vi "LEP_RV_BuildSettingsDefault.vi"(3 "error in (no error)":errorcluster) -> (0 "error out":errorcluster, 1 "Default Values":refnum<vi>[](array[refnum]), 2 "Attribute Name":string[](array[string]))   [LabVIEW 2011]
doc: "Sets the default project settings for new LabVIEW Embedded Projects."
uses:
  LEP_RV_Config.ctl
panel:
  in  "Default":T1={"Enable debugging"=TRUE, "Debug Options"=0, "Use stack variables"=FALSE, "Generate serial only"=FALSE, "Generate guard code"=TRUE, "Generate Integer Only"=FALSE, "Generate C Function Calls"=FALSE, "ExpressionFolding"=FALSE, "Constant Allocation"=0, "Constant Deallocation"=0, "Build Specification ID"="", "Preprocessor symbols (define)"="", "Compiler Flags"="", "Linker Flags"="", "Mode"=1, "Optimization"=2, "Optimize for time"=FALSE, "Enable cross-module optimization"=TRUE, "Include paths"=[], "Optimize heap size"=TRUE, "Use MicroLib"=FALSE, "Debug Mode"=2, "Enable profile information"=FALSE, "Host name"="board", "Use DHCP"=TRUE, "IP address"="0.0.0.0", "Subnet mask"="0.0.0.0", "Gateway"="0.0.0.0", "Primary DNS"="0.0.0.0", "Secondary DNS"="0.0.0.0", "MAC in target memory"=TRUE, "MAC address"="", "Console output"=0, "Target serial port"=0} {"Constant Deallocation" items=["Out of Scope", "VI End", "Application End"]; "Constant Allocation" items=["First Use", "Containing Loop", "VI Initialization", "Application Initialization"]; "Target serial port" items=["0", "1", "2", "3"]; "Console output" items=["Processor status window", "Serial port"]; "Optimization" items=["Level 0 (-O0)", "Level 1 (-O1)", "Level 2 (-O2)", "Level 3 (-O3)"]; "Mode" items=["ARM-Mode", "Thumb-Mode"]; "Debug Options" items=["Use ULINK Debugger", "Use Simulator"]; "Debug Mode" items=["Instrumented (serial port)", "Instrumented (TCP/IP)", "Non-instrumented (JTAG/USB)"]}
  out "Default":T1={"Enable debugging"=TRUE, "Debug Options"=0, "Use stack variables"=FALSE, "Generate serial only"=FALSE, "Generate guard code"=TRUE, "Generate Integer Only"=FALSE, "Generate C Function Calls"=FALSE, "ExpressionFolding"=FALSE, "Constant Allocation"=0, "Constant Deallocation"=0, "Build Specification ID"="", "Preprocessor symbols (define)"="", "Compiler Flags"="", "Linker Flags"="", "Mode"=1, "Optimization"=2, "Optimize for time"=FALSE, "Enable cross-module optimization"=TRUE, "Include paths"=[], "Optimize heap size"=TRUE, "Use MicroLib"=FALSE, "Debug Mode"=2, "Enable profile information"=FALSE, "Host name"="board", "Use DHCP"=TRUE, "IP address"="0.0.0.0", "Subnet mask"="0.0.0.0", "Gateway"="0.0.0.0", "Primary DNS"="0.0.0.0", "Secondary DNS"="0.0.0.0", "MAC in target memory"=TRUE, "MAC address"="", "Console output"=0, "Target serial port"=1} {"Constant Deallocation" items=["Out of Scope", "VI End", "Application End"]; "Constant Allocation" items=["First Use", "Containing Loop", "VI Initialization", "Application Initialization"]; "Target serial port" items=["0", "1", "2", "3"]; "Console output" items=["Processor status window", "Serial port"]; "Optimization" items=["Level 0 (-O0)", "Level 1 (-O1)", "Level 2 (-O2)", "Level 3 (-O3)"]; "Mode" items=["ARM-Mode", "Thumb-Mode"]; "Debug Options" items=["Use ULINK Debugger", "Use Simulator"]; "Debug Mode" items=["Instrumented (serial port)", "Instrumented (TCP/IP)", "Non-instrumented (JTAG/USB)"]}
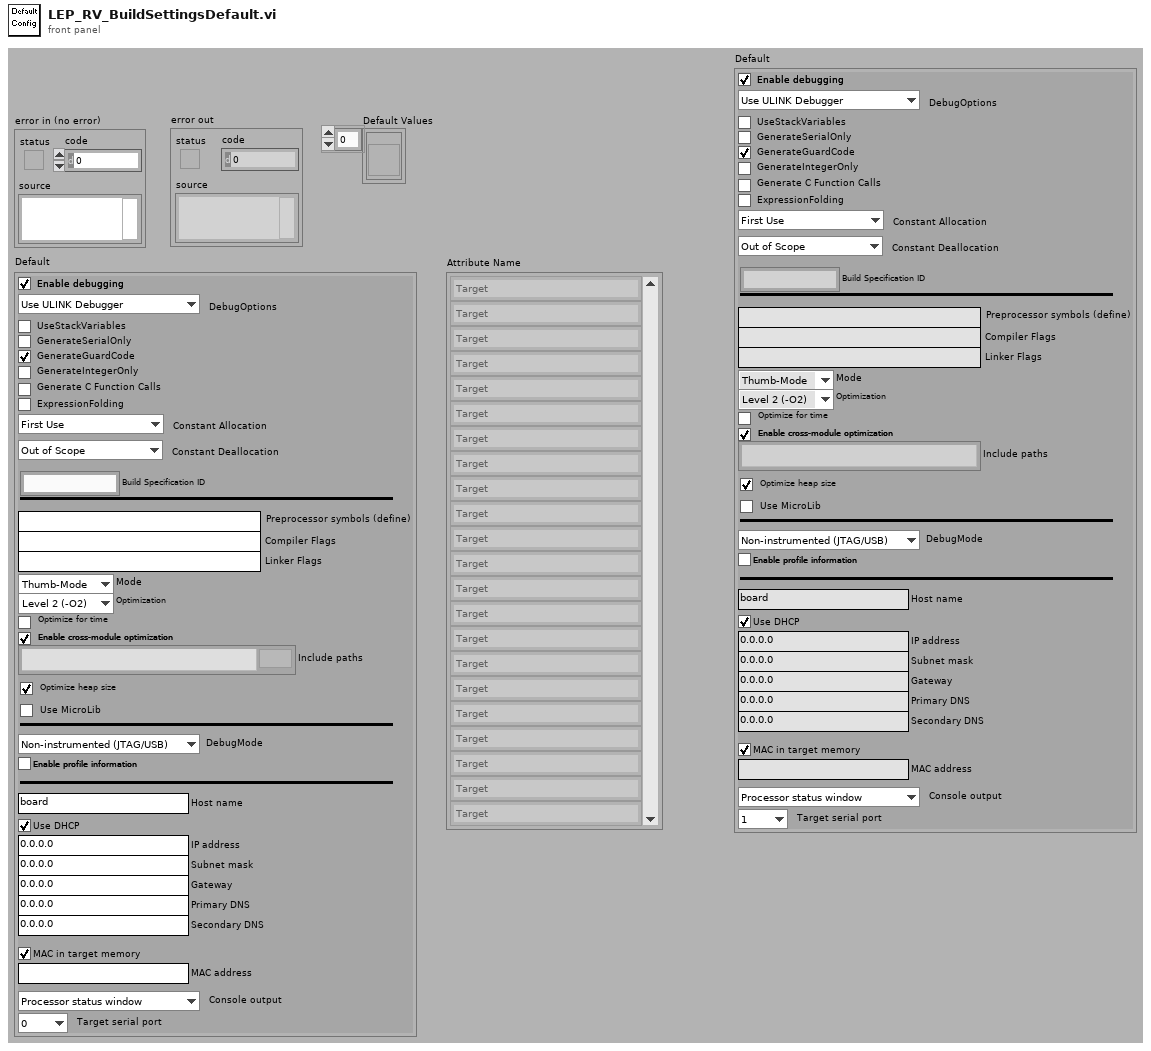
[diagram p1: front panel]
types:
  T1 = typedef "LEP_RV_Config.ctl" = cluster{"Enable debugging":bool, "Debug Options":u16, "Use stack variables":bool, "Generate serial only":bool, "Generate guard code":bool, "Generate Integer Only":bool, "Generate C Function Calls":bool, "ExpressionFolding":bool, "Constant Allocation":u16, "Constant Deallocation":u16, "Build Specification ID":string, "Preprocessor symbols (define)":string, "Compiler Flags":string, "Linker Flags":string, "Mode":u16, "Optimization":u16, "Optimize for time":bool, "Enable cross-module optimization":bool, "Include paths":path[], "Optimize heap size":bool, "Use MicroLib":bool, "Debug Mode":u16, "Enable profile information":bool, "Host name":string, "Use DHCP":bool, "IP address":string, "Subnet mask":string, "Gateway":string, "Primary DNS":string, "Secondary DNS":string, "MAC in target memory":bool, "MAC address":string, "Console output":u16, "Target serial port":u16}
  T2 = cluster{"Item URL":string, "Item ID":string, "Item Index":i32, "Specific Type":string}
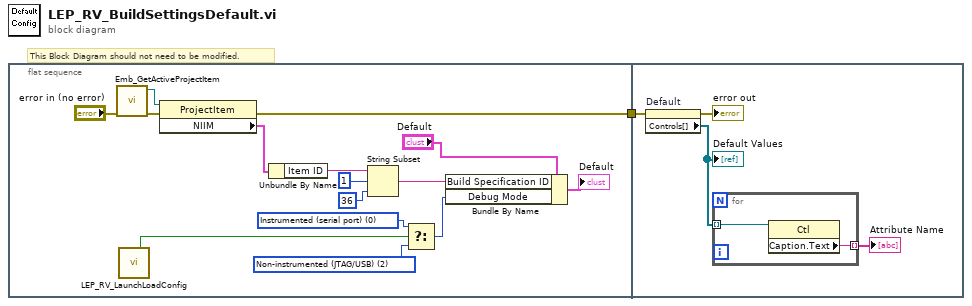
[diagram p0: block diagram]
diagram:
  # "This Block Diagram should not need to be modified."
  n1 = flat-sequence {
    tunnel: [w13] -> w1
    tunnel: w1 -> [w17]
    frame #0 {
      w4 = u16 2 items=["Instrumented (serial port)", "Instrumented (TCP/IP)", "Non-instrumented (JTAG/USB)"] ("Debug Mode")
      w5 = u16 0 items=["Instrumented (serial port)", "Instrumented (TCP/IP)", "Non-instrumented (JTAG/USB)"] ("Debug Mode")
      n2 = call "Emb_GetActiveProjectItem.vi"("error in (no error)"="error in (no error)") -> ("error out"=w14:errorcluster, "ProjectItem Refnum"=w11:refnum<vi>)  [unwired: 9 out]
      n3 = call "LEP_RV_LaunchLoadConfig.vi"() -> ("Connect to a network compile server"=w2:bool)  [unwired: 8 in, 7 out]
      n4 = property class="ProjectItem"(reference=w11, error in=w14) -> (error out=w13:errorcluster, "NIIM"=w12:T2)  [unwired: 1 out]
      n5 = Unbundle By Name(w12) -> ("Item ID"=w9:string)
      n6 = String Subset(string=w9, offset (0)=1, length (rest)=36 ("length (rest)")) -> (substring=w6:string)
      n7 = Select(t=w5, s=w2, f=w4) -> (s? t:f=w3:u16)
      n8 = Bundle By Name(cluster="Default", "Build Specification ID"=w6, "Debug Mode"=w3) -> (→"Default":T1)
    }
    frame #1 {
      n9 = property on="Default" class="Clust (strict)"(error in=w17) -> (error out=→"error out":errorcluster, "Controls[]"=w19:refnum<vi>[])  [unwired: 1 in, 1 out]
      "Default Values" <- w19
      n10 = for {
        tunnel: w19 -> [w22] mode=indexing
        tunnel: [w21] -> w18 mode=indexing
        n11 = property class="Ctl"(reference=w22) -> ("Caption.Text"=w21:string)  [unwired: 1 in, 2 out]
      }
      "Attribute Name" <- w18
    }
  }
